vi "Global Optimization_Circle_Objective Function.vi"(9 "output selector":T1, 10 "data":variant, 11 "X":dbl[](array[numeric])) -> (0 "error out":errorcluster, 1 "Inequality Constraints":dbl[](array[numeric]), 2 "Equality Constraints":dbl[](array[numeric]), 3 "Objective Functions":dbl[](array[numeric]))   [LabVIEW 2017]
uses:
  <vilib>/gmath/NumericalOptimization/cno_output select.ctl
  <vilib>/gmath/NI_Gmath.lvlib
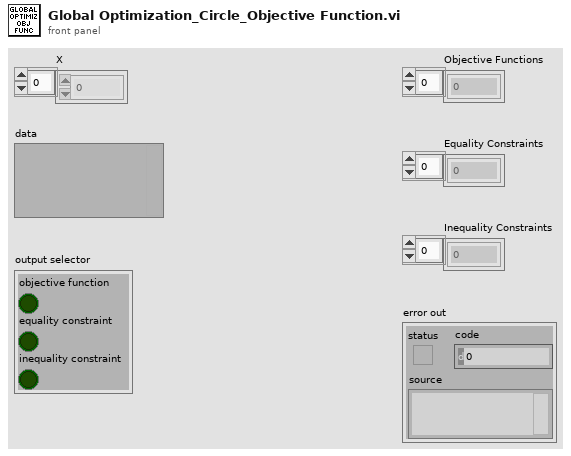
[diagram p1: front panel]
types:
  T1 = typedef "NI_Gmath.lvlib/cno_output select.ctl" = cluster{"objective function":bool, "equality constraint":bool, "inequality constraint":bool}
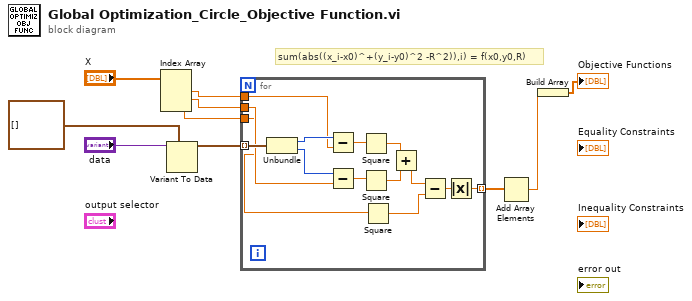
[diagram p0: block diagram]
diagram:
  # "sum(abs((x_i-x0)^+(y_i-y0)^2 -R^2)),i) = f(x0,y0,R)"
  n1 = Index Array(array="X") -> (element #1=w6:dbl, element #2=w5:dbl, element #3=w4:dbl)  [unwired: 3 in]
  n2 = Variant To Data(type=cluster{i32, i32}[] [], Variant="data") -> (data=w7:cluster{i32, i32}[])  [unwired: 1 in, 1 out]
  n3 = for {
    tunnel: w7 -> [w24] mode=indexing
    tunnel: w6 -> [w21]
    tunnel: w5 -> [w20]
    tunnel: w4 -> [w15]
    tunnel: [w11] -> w3 mode=indexing
    n4 = Unbundle(w24) -> (w23:i32, w22:i32)
    n5 = Subtract(x=w23, y=w21) -> (x-y=w19:dbl)
    n6 = Subtract(x=w22, y=w20) -> (x-y=w18:dbl)
    n7 = Square(x=w19) -> (x^2=w17:dbl)
    n8 = Square(x=w18) -> (x^2=w16:dbl)
    n9 = Square(x=w15) -> (x^2=w13:dbl)
    n10 = Add(x=w17, y=w16) -> (x+y=w14:dbl)
    n11 = Subtract(x=w14, y=w13) -> (x-y=w12:dbl)
    n12 = Absolute Value(x=w12) -> (abs(x)=w11:dbl)
  }
  n13 = Add Array Elements(numeric array=w3) -> (sum=w2:dbl)
  n14 = Build Array(w2) -> (→"Objective Functions":dbl[])
